vi "Setup encoder in.vi"(8 "error in (no error)":errorcluster, 10 "Run info in":T1, 11 "Sampling info in":T2 {"Channels"."Hi cutoff" items=["500"=500.0, "1k"=1000.0, "5k"=5000.0, "10k"=10000.0, "20k"=20000.0]; "Channels"."Lo cutoff" items=["0.1"=0.1, "1"=1.0, "10"=10.0, "100"=100.0, "300"=300.0]; "Channels"."Gain" items=["x100"=100, "x1000"=1000, "x10000"=10000]}) -> (0 "error out":errorcluster, 2 "Run info":T1, 3 "Sampling info out":T2 {"Channels"."Hi cutoff" items=["500"=500.0, "1k"=1000.0, "5k"=5000.0, "10k"=10000.0, "20k"=20000.0]; "Channels"."Lo cutoff" items=["0.1"=0.1, "1"=1.0, "10"=10.0, "100"=100.0, "300"=300.0]; "Channels"."Gain" items=["x100"=100, "x1000"=1000, "x10000"=10000]})   [LabVIEW 2012]
uses:
  Sampling info.ctl
  Channel.ctl
  Run info.ctl
  <vilib>/DAQmx/create/channels.llb/DAQmx Create Channel (CI-Position-Angular Encoder).vi
  <vilib>/DAQmx/configure/timing.llb/DAQmx Timing (Sample Clock).vi
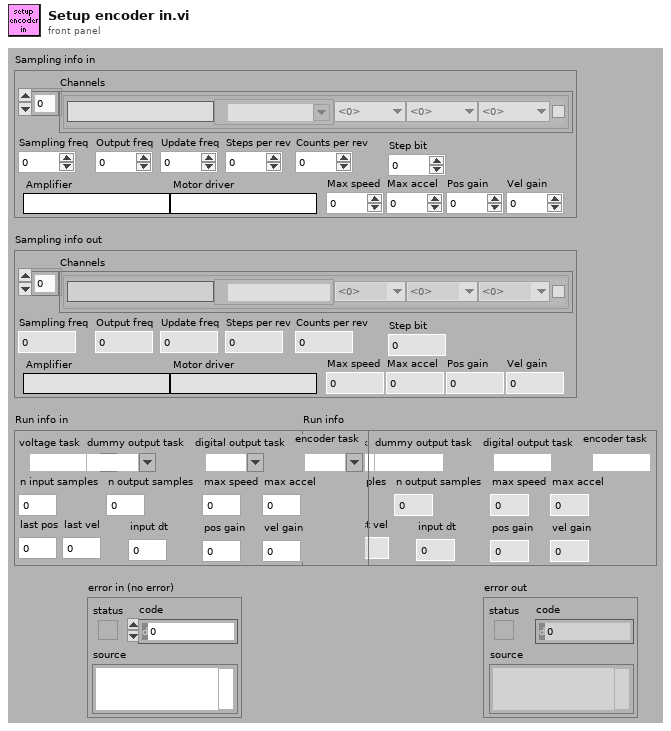
[diagram p1: front panel]
types:
  T1 = typedef "Run info.ctl" = cluster{"voltage task":refnum<k21>, "dummy output task":refnum<k21>, "digital output task":refnum<k21>, "encoder task":refnum<k21>, "n input samples":i32, "n output samples":i32, "max speed":dbl, "max accel":dbl, "last pos":dbl, "last vel":dbl, "pos gain":dbl, "vel gain":dbl, "input dt":dbl}
  T2 = typedef "Sampling info.ctl" = cluster{"Channels":T3[], "Sampling freq":i32, "Output freq":i32, "Update freq":i32, "Steps per rev":i32, "Counts per rev":i32, "Amplifier":string, "Motor driver":string, "Step bit":u8, "Max speed":dbl, "Max accel":dbl, "Pos gain":dbl, "Vel gain":dbl}
  T3 = typedef "Channel.ctl" = cluster{"Name":string, "Chan":tag, "Gain":u16, "Lo cutoff":dbl, "Hi cutoff":dbl, "Notch":bool}
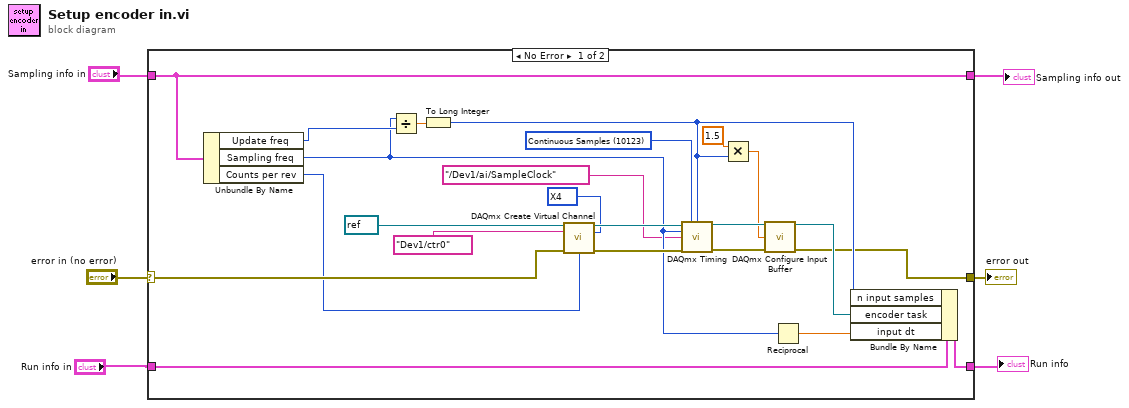
[diagram p0: block diagram]
diagram:
  n1 = case shown="No Error" "error in (no error)" {
    selector: "error in (no error)" -> [w27 w31]
    tunnel: [w26 w30] -> w2
    tunnel: [w13 w31] -> w5
    tunnel: [w28 w32] -> w1
    tunnel: "Sampling info in" -> [w28 w32]
    tunnel: "Run info in" -> [w25 w30]
    frame No Error {
      w8 = 10092 items=["X1"=10090, "X2"=10091, "X4"=10092, "Two Pulse Counting"=10313] ("decoding type")
      w22 = 10123 items=["Finite Samples"=10178, "Continuous Samples"=10123, "Hardware Timed Single Point"=12522] ("sample mode")
      n2 = Unbundle By Name(w28) -> ("Update freq"=w21:i32, "Sampling freq"=w12:i32, "Counts per rev"=w9:i32)
      n3 = Divide(x=w12, y=w21) -> (x/y=w20:dbl)
      n4 = To Long Integer(number=w20) -> (32bit integer=w16:i32)
      n5 = call-poly <vilib>:"DAQmx Create Virtual Channel.vi"("task in"=refnum<k21> refnum ("task out"), "counter"=tag "Dev1/ctr0", "decoding type"=w8, "error in"=w27, "pulses per revolution"=w9) -> ("task out"=w24:refnum<k21>, "error out"=w23:errorcluster)  [unwired: 7 in, 2 out]
      n6 = call-poly <vilib>:"DAQmx Timing.vi"("task/channels in"=w24, "sample mode"=w22, "samples per channel"=w16, "rate"=w12, "source"=tag "/Dev1/ai/SampleClock", "error in"=w23) -> ("task out"=w19:refnum<k21>, "error out"=w18:errorcluster)  [unwired: 8 in]
      n7 = Multiply(x=1.5, y=w16) -> (x*y=w15:dbl)
      n8 = call <vilib>:"DAQmx Configure Input Buffer.vi"("task/channels in"=w19, "buffer size (in samples per channel)"=w15, "error in"=w18) -> ("task out"=w14:refnum<k21>, "error out"=w13:errorcluster)  [unwired: 11 in]
      n9 = Reciprocal(x=w12) -> (1/x=w11:dbl)
      n10 = Bundle By Name(cluster=w25, "n input samples"=w16, "encoder task"=w14, "input dt"=w11) -> (w26:T1)
    }
    frame Error {
    }
  }
  "error out" <- w5
  "Run info" <- w2
  "Sampling info out" <- w1
